vi "Power Output PWM Calibration.vi"(6 "Drv Refnum":T1, 8 "error in (no error)":errorcluster, 10 "Force Calibration (F)":bool, 11 "Seq Count":u32) -> (0 "error out":errorcluster, 2 "Next Action":string, 3 "Calibrated?":T2, 4 "dup Drv Refnum":T1)   [LabVIEW 2011]
uses:
  drivers/PWM/PWM Normalization State.ctl
  drivers/PWM/PWM Driver Ref.ctl
  drivers/Calibration INI File Command.ctl
  drivers/Calibration INI File Driver.ctl
  drivers/PWM/PWM Command.ctl
  drivers/PWM/PWM Calibration INI File.vi
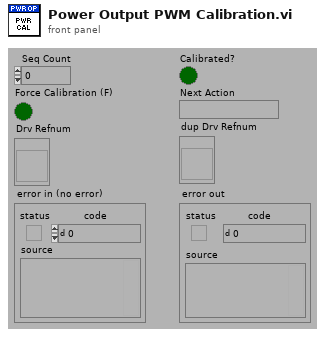
[diagram p1: front panel]
types:
  T1 = typedef "PWM Driver Ref.ctl" = refnum<vi>
  T2 = typedef "PWM Normalization State.ctl" = bool
  T3 = typedef "Calibration INI File Driver.ctl" = enum16{"ATT", "DMM", "IMP", "PFE", "PIM", "PWM", "SNA", "SWI", "VNA"}
  T4 = typedef "Calibration INI File Command.ctl" = enum16{"Read", "Write", "Clear"}
  T5 = typedef "PWM Command.ctl" = enum16{"LOAD", "INITIALIZE", "PRESET", "GET STIMULUS", "SET STIMULUS", "MEASURE", "RELEASE", "UNLOAD", "GET CALIBRATION", "CALIBRATE"}
  T6 = typedef "Power Output Dialog Response.ctl" = enum16{"Continue", "Calibrate", "Ignore", "Abort", "Abort All"}
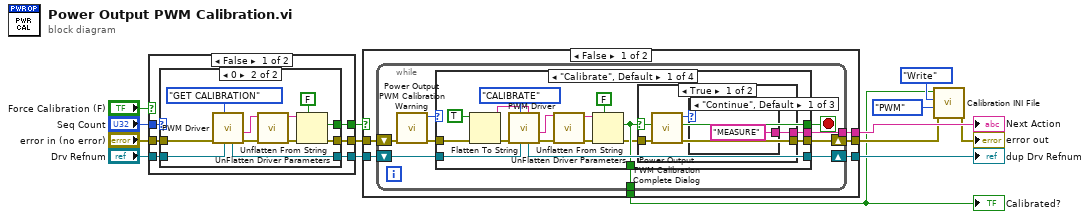
[diagram p0: block diagram]
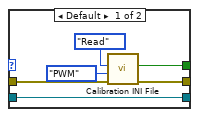
[diagram p2: hidden frame]
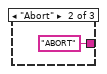
[diagram p4: hidden frame]
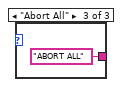
[diagram p5: hidden frame]
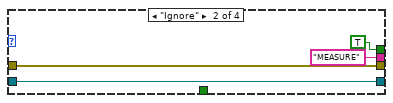
[diagram p7: hidden frame]
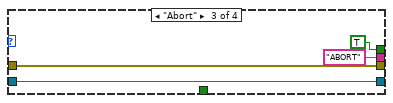
[diagram p8: hidden frame]
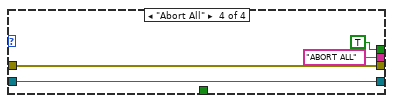
[diagram p9: hidden frame]
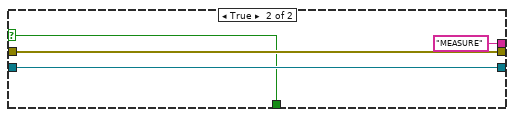
[diagram p10: hidden frame]
diagram:
  n1 = case shown="False" "Force Calibration (F)" {
    tunnel: "Seq Count" -> [w20 _]
    tunnel: [w19 _] -> w13
    tunnel: [w18 w39] -> w12
    tunnel: [w17 w38] -> w11
    tunnel: "Drv Refnum" -> [w16 w38]
    tunnel: "error in (no error)" -> [w15 w39]
    frame False {
      n2 = case shown="0" w20 {
        tunnel: w15 -> [w24 w36]
        tunnel: w16 -> [w22 w35]
        tunnel: [w22 w34] -> w17
        tunnel: [w23 w31] -> w18
        tunnel: [w21 w27] -> w19
        frame Default {
          n3 = call-poly "Calibration INI File.vi"("error in (no error)"=w24, "Driver"=Calibration_INI_File_Driver."PWM", "Operation"=Calibration_INI_File_Command."Read") -> ("error out"=w23:errorcluster, "Calibration Out"=w21:T2)  [unwired: 7 in]
        }
        frame 0 {
          n4 = call "PWM Driver.vi"("Drv Refnum"=w35, "PWM Command"=PWM_Command."GET CALIBRATION" ("DMM Command"), "error in (no error)"=w36) -> ("error out"=w33:errorcluster, "Variant Output"=w30:string, "dup Drv Refnum"=w34:T1)  [unwired: 5 in, 1 out]
          n5 = call "UnFlatten Driver Parameters.vi"("error in (no error)"=w33, "Flattened Driver Parameters with Version (\"\")"=w30) -> ("error out"=w32:errorcluster, "Flat Driver Parameters"=w29:string)  [unwired: 3 in, 1 out]
          n6 = Unflatten From String(type=T2 FALSE ("Normalized?"), binary string=w29, error in (no error)=w32) -> (value=w27:T2, error out=w31:errorcluster)  [unwired: 3 out]
        }
      }
    }
    frame True {
    }
  }
  n7 = case shown="False" w13 {
    selector: w13 -> [_ w91]
    tunnel: [w45 w94] -> w7
    tunnel: [w44 w93] -> w3
    tunnel: [w43 "MEASURE"] -> w10
    tunnel: w11 -> [w42 w94]
    tunnel: w12 -> [w41 w93]
    tunnel: [w40 w91] -> w2
    frame False {
      n8 = while {
        shift-right: [w52] -> w44
        shift-left: w41 -> [w51]
        shift-right: [w53] -> w45
        shift-left: w42 -> [w54]
        tunnel: [w47] -> w43
        tunnel: [w46] -> w40
        stop <- w48 stop-if-true
        n9 = call "Power Output PWM Calibration Warning.vi"("error in (no error)"=w51) -> ("error out"=w50:errorcluster, "Choice"=w49:T6)  [unwired: 9 in]
        n10 = case shown="\"Calibrate\", Default" w49 {
          tunnel: w54 -> [w69 w82 w86 w90]
          tunnel: [w68 w82 w86 w90] -> w53
          tunnel: [w55 w81 w85 w89] -> w52
          tunnel: w50 -> [w64 w81 w85 w89]
          tunnel: [w57 TRUE ("replace all? (F)") TRUE ("replace all? (F)") TRUE ("replace all? (F)")] -> w48
          tunnel: [w63 "MEASURE" "ABORT" "ABORT ALL"] -> w47
          tunnel: [w57 _ _ _] -> w46
          frame "Calibrate", Default {
            n11 = Flatten To String(anything=T2 TRUE, error in (no error)=w64) -> (data string=w65:string, error out=w66:errorcluster)  [unwired: 2 in, 1 out]
            n12 = call "PWM Driver.vi"("PWM Configuration (\"\")"=w65, "Drv Refnum"=w69, "PWM Command"=PWM_Command."CALIBRATE" ("DMM Command"), "error in (no error)"=w66) -> ("error out"=w59:errorcluster, "Variant Output"=w58:string, "dup Drv Refnum"=w68:T1)  [unwired: 4 in, 1 out]
            n13 = call "UnFlatten Driver Parameters.vi"("error in (no error)"=w59, "Flattened Driver Parameters with Version (\"\")"=w58) -> ("error out"=w60:errorcluster, "Flat Driver Parameters"=w61:string)  [unwired: 3 in, 1 out]
            n14 = Unflatten From String(type=T2 FALSE ("Normalized?"), binary string=w61, error in (no error)=w60) -> (value=w57:T2, error out=w56:errorcluster)  [unwired: 3 out]
            n15 = case shown="True" w57 {
              tunnel: [w74 _] -> w63
              tunnel: w56 -> [w73 w78]
              tunnel: [w72 w78] -> w55
              frame True {
                n16 = call "Power Output PWM Calibration Complete Dialog.vi"("error in (no error)"=w73) -> ("error out"=w72:errorcluster, "Choice"=w71:T6)  [unwired: 9 in]
                n17 = case shown="\"Continue\", Default" w71 {
                  tunnel: ["MEASURE" "ABORT" "ABORT ALL"] -> w74
                  frame "Continue", Default {
                  }
                  frame "Abort" {
                  }
                  frame "Abort All" {
                  }
                }
              }
              frame False {
              }
            }
          }
          frame "Ignore" {
          }
          frame "Abort" {
          }
          frame "Abort All" {
          }
        }
      }
    }
    frame True {
    }
  }
  "Calibrated?" <- w2
  "Next Action" <- w10
  "dup Drv Refnum" <- w7
  n18 = call-poly "Calibration INI File.vi"("error in (no error)"=w3, "Driver"=Calibration_INI_File_Driver."PWM", "Operation"=Calibration_INI_File_Command."Write", "Calibration In"=w2) -> ("error out"=→"error out":errorcluster)  [unwired: 6 in, 1 out]
